vi "VSG25_SelectDevice.vi"(2 "ErrorIn":errorcluster, 3 "AutoSel":bool) -> (0 "ErrorOut":errorcluster, 1 "deviceHandle":i32)   [LabVIEW 2014]
uses:
  sg_lib/VSG25A.lvlib
panel:
  in  "Cancel Button":bool
  in  "Open Button":bool
  in  "Available Devices":string(combo)
  out "numOfDevices":i32
  out "deviceList":i32[](array[numeric])
  out "API Version:":string
  # "Select VSG25 Device to Open"
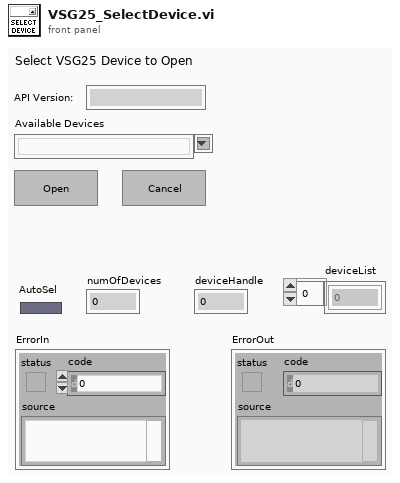
[diagram p1: front panel]
types:
  T1 = enum32{"Bad", "Idle", "Run top level", "Running"}
  T2 = enum16{"GetDevices", "ProcEvent", "SelectDevice", "Exit"}
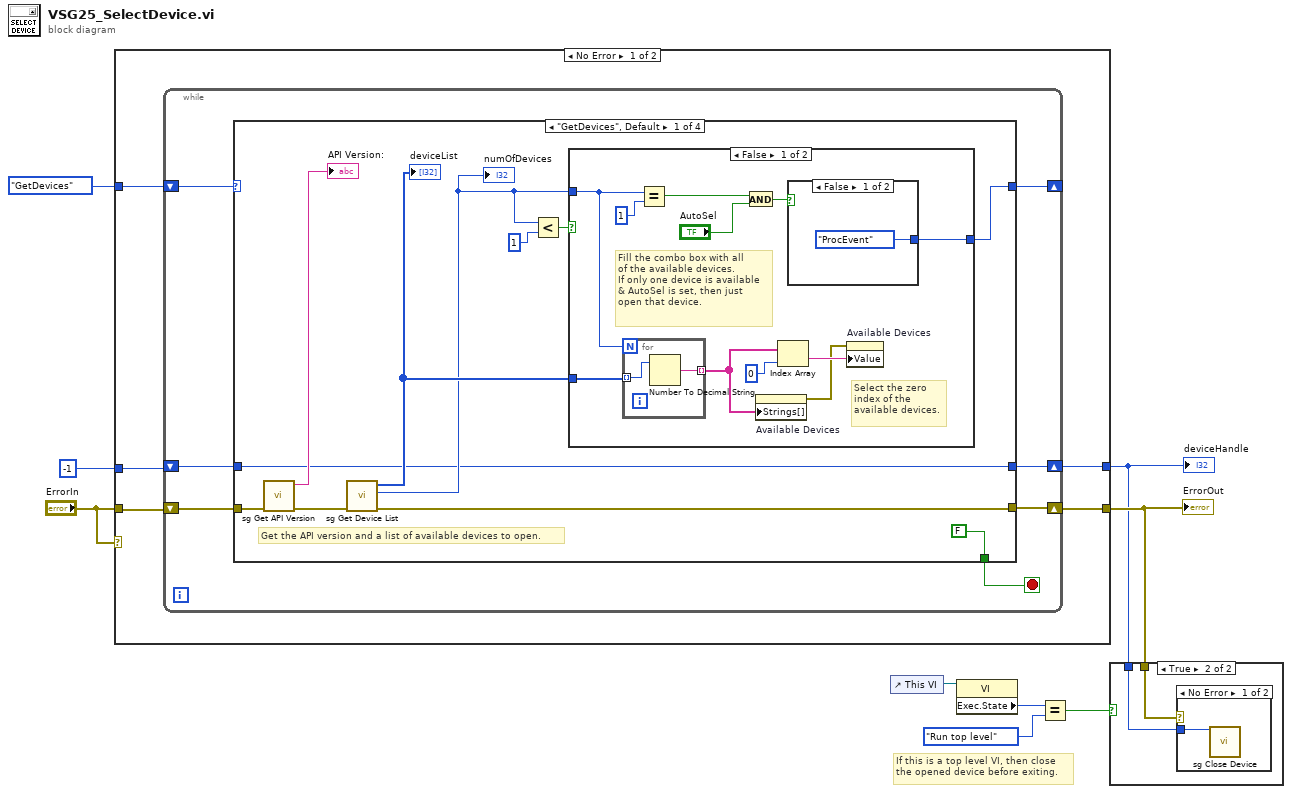
[diagram p0: block diagram]
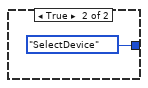
[diagram p4: hidden frame]
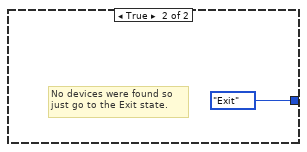
[diagram p5: hidden frame]
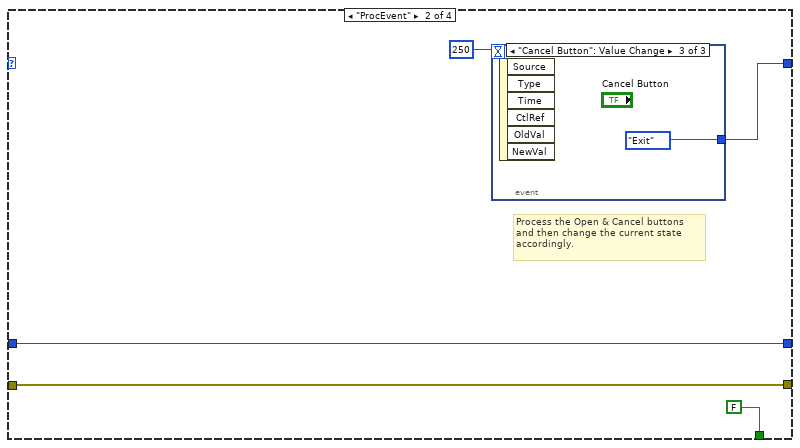
[diagram p6: hidden frame]
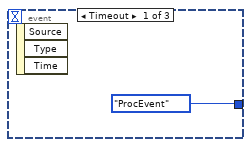
[diagram p7: hidden frame]
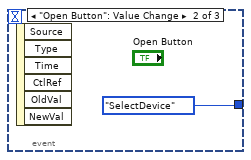
[diagram p8: hidden frame]
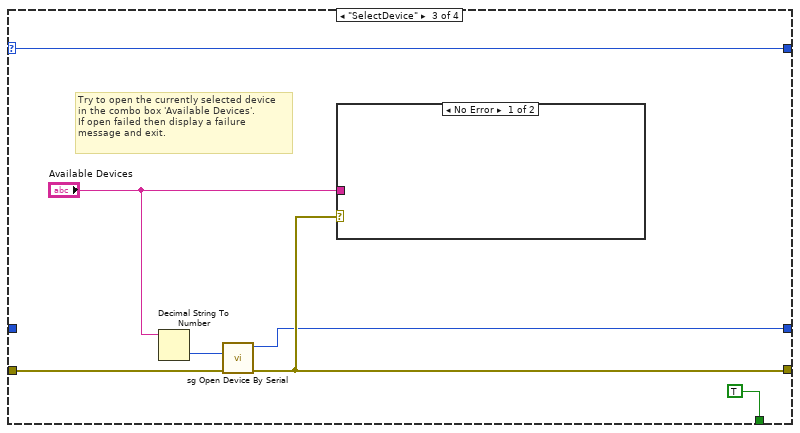
[diagram p9: hidden frame]
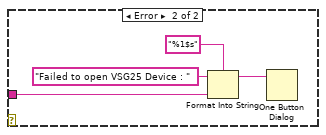
[diagram p10: hidden frame]
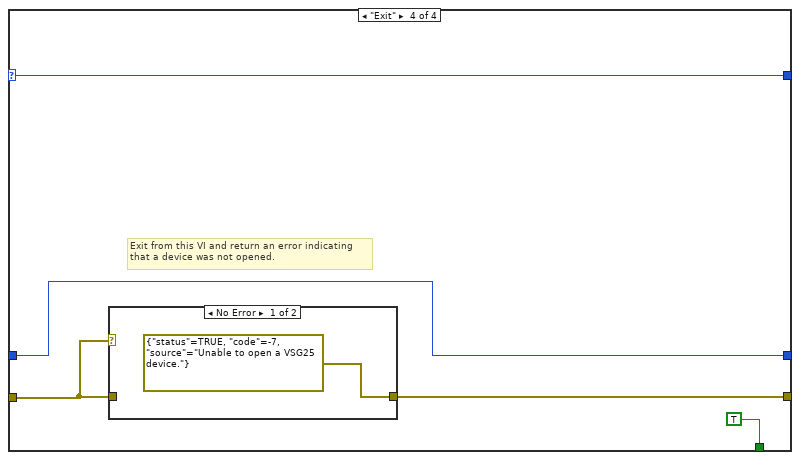
[diagram p11: hidden frame]
diagram:
  # "If this is a top level VI, then close\nthe opened device before exiting."
  n1 = case shown="No Error" "ErrorIn" {
    tunnel: "ErrorIn" -> [w14 w76]
    tunnel: T2."GetDevices" -> [w13 _]
    tunnel: [w12 w76] -> w7
    tunnel: [w11 w75] -> w6
    tunnel: -1 ("device out") -> [w10 w75]
    frame No Error {
      n2 = while {
        shift-right: [w20] -> _
        shift-left: w13 -> [w21]
        shift-right: [w17] -> w12
        shift-left: w14 -> [w18]
        shift-right: [w16] -> w11
        shift-left: w10 -> [w15]
        stop <- w19 stop-if-true
        n3 = case shown="\"GetDevices\", Default" w21 {
          selector: w21 -> [_ _ w57 w72]
          tunnel: [w27 w51 w57 w72] -> w20
          tunnel: [FALSE FALSE TRUE TRUE] -> w19
          tunnel: w18 -> [w24 w50 w61 w70]
          tunnel: [w23 w50 w59 w69] -> w17
          tunnel: [w22 w49 w58 w68] -> w16
          tunnel: w15 -> [w22 w49 _ w68]
          frame "GetDevices", Default {
            # "Get the API version and a list of available devices to open."
            n4 = call "sg Get API Version.vi"("error in (no error)"=w24) -> ("error out"=w29:errorcluster, "function return"=→"API Version:":string)  [unwired: 9 in]
            n5 = call "sg Get Device List.vi"("error in (no error)"=w29) -> ("error out"=w23:errorcluster, "length out"=w31:i32, "deviceList out"=w32:i32[])  [unwired: 7 in, 1 out]
            "deviceList" <- w32
            "numOfDevices" <- w31
            n6 = Less?(x=w31, y=1) -> (x < y?=w30:bool)
            n7 = case shown="False" w30 {
              tunnel: w31 -> [w38 _]
              tunnel: w32 -> [w43 _]
              tunnel: [w42 T2."Exit"] -> w27
              frame False {
                # "Select the zero\nindex of the \navailable devices."
                # "Fill the combo box with all\nof the available devices. \nIf only one device is available\n& AutoSel is set, then just \nopen that device."
                n8 = for {
                  N: w38 -> [_]
                  tunnel: [w45] -> w41 mode=indexing
                  tunnel: w43 -> [w44] mode=indexing
                  n9 = Number To Decimal String(number=w44) -> (decimal integer string=w45:string)  [unwired: 1 in]
                }
                n10 = Equal?(x=w38, y=1) -> (x = y?=w34:bool)
                n11 = And(x=w34, y="AutoSel") -> (x .and. y?=w35:bool)
                n12 = property on="Available Devices" class="CmbBox"("Strings[]"=w41) -> (error out=w36:errorcluster)  [unwired: 2 in, 1 out]
                n13 = Index Array(array=w41, index=0) -> (element=w39:string)
                n14 = case shown="False" w35 {
                  tunnel: [T2."ProcEvent" T2."SelectDevice"] -> w42
                  frame False {
                  }
                  frame True {
                  }
                }
                n15 = property on="Available Devices" class="CmbBox"(error in=w36, "Value"=w39) -> ()  [unwired: 1 in, 2 out]
              }
              frame True {
                # "No devices were found so\njust go to the Exit state."
              }
            }
          }
          frame "ProcEvent" {
            # "Process the Open & Cancel buttons\nand then change the current state \naccordingly."
            n16 = event shown="[2] \"Cancel Button\": Value Change" {
              selector: _ -> [_ _ _]
              dyn-events: _ -> [_ _ _]
              timeout: 250 -> [_ _ _]
              tunnel: [T2."ProcEvent" T2."SelectDevice" T2."Exit"] -> w51
              event Timeout {
                n17 = event-data() -> ()  [unwired: 1 in, 3 out]
              }
              event "Open Button": Value Change {
                n18 = event-data() -> ()  [unwired: 1 in, 6 out]
              }
              event "Cancel Button": Value Change {
                n19 = event-data() -> ()  [unwired: 1 in, 6 out]
              }
            }
          }
          frame "SelectDevice" {
            # "Try to open the currently selected device\nin the combo box 'Available Devices'.\nIf open failed then display a failure\nmessage and exit."
            n20 = Decimal String To Number(string="Available Devices") -> (number=w62:i32)  [unwired: 2 in, 1 out]
            n21 = call "sg Open Device By Serial.vi"("error in (no error)"=w61, "serialNumber"=w62) -> ("error out"=w59:errorcluster, "device out"=w58:i32)  [unwired: 7 in, 1 out]
            n22 = case shown="No Error" w59 {
              tunnel: "Available Devices" -> [_ w64]
              frame No Error {
              }
              frame Error {
                n23 = Format Into String(format string="%1$s", initial string="Failed to open VSG25 Device : ", w64) -> (resulting string=w67:string)  [unwired: 1 in, 1 out]
                n24 = One Button Dialog(message=w67) -> ()  [unwired: 1 in, 1 out]
              }
            }
          }
          frame "Exit" {
            # "Exit from this VI and return an error indicating\nthat a device was not opened."
            n25 = case shown="No Error" w70 {
              tunnel: w70 -> [_ w74]
              tunnel: [errorcluster {"status"=TRUE, "code"=-7, "source"="Unable to open a VSG25 device."} ("error constant") w74] -> w69
              frame No Error {
              }
              frame Error {
              }
            }
          }
        }
      }
    }
    frame Error {
    }
  }
  "ErrorOut" <- w7
  "deviceHandle" <- w6
  n26 = control-ref of="This VI"() -> (w4:refnum<vi>)
  n27 = property class="VI"(reference=w4) -> ("Exec.State"=w3:T1)  [unwired: 1 in, 2 out]
  n28 = Equal?(x=w3, y=T1."Run top level" ("Execution:State 2")) -> (x = y?=w1:bool)
  n29 = case shown="True" w1 {
    tunnel: w7 -> [_ w78]
    tunnel: w6 -> [_ w77]
    frame False {
    }
    frame True {
      n30 = case shown="No Error" w78 {
        tunnel: w77 -> [w79 _]
        frame No Error {
          n31 = call "sg Close Device.vi"("device"=w79) -> ()  [unwired: 9 in, 2 out]
        }
        frame Error {
        }
      }
    }
  }
